vi "SwissSPAD Live_Create HDF5 File.vi"(8 "error in (no error)":errorcluster, 10 "Current Acquisition":i32, 11 "Current Data Set":i32) -> (0 "Error Out":errorcluster, 1 "Notebook Message":string, 2 "# Image Sets":u32, 3 "# Datasets in Series":i32, 5 "Gate Image Data Q Name":string)   [LabVIEW 2021]
uses:
  SwissSPAD Live_Settings List.ctl
  SwissSPAD Live_File Information.ctl
  <vilib>/addons/h5labview2/file/H5Fmode.ctl
  SwissSPAD Live_SSx PCB Version.ctl
  SwissSPAD Live_SS2 DAQ Parameters 3.ctl
  SwissSPAD Live_SS2 Gate Definition.ctl
  SwissSPAD Live_SS3 DAQ Parameters.ctl
  SwissSPAD Live_SS3 Gate Definition.ctl
  SS3 Gate Width Definition Mode.ctl
  <vilib>/Utility/error.llb/Error Cluster From Error Code.vi
  SwissSPAD Live_Globals.vi
  <vilib>/ErrorRing/Error Ring.xnode
  <vilib>/addons/h5labview2/file/H5F.lvlib
  Variant/Variant to Data/Variant to Data.lvlib
panel:
  out "File Folder":path
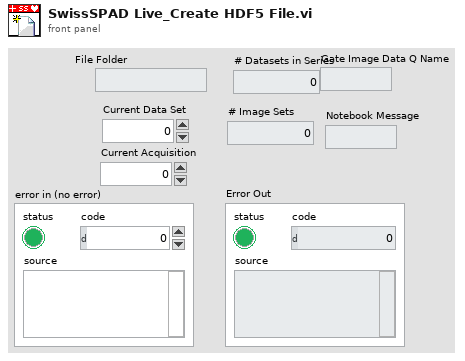
[diagram p1: front panel]
types:
  T1 = typedef "SwissSPAD Live_Settings List.ctl" = enum16{"FPGA:Bottom Half", "FPGA:Top Half", "FPGA:Bottom Bitfile Path", "FPGA:Top Bitfile Path", "FPGA:Bottom Bitstream Version", "FPGA:Top Bitstream Version", "FPGA:Auto Reset FPGA", "FPGA:Bottom FPGA Serial Number", "FPGA:Top FPGA Serial Number", "FPGA:Detector PCB Version", "Acquisition Parameters:Microlens", "Acquisition Parameters:SS2 DAQ Parameters", "Acquisition Parameters:Gate Configuration Array", "Acquisition Parameters:SS3 DAQ Parameters", "Acquisition Parameters:Buffer Size (# 8-bit Gates)", "File Information:File Information", "File Information:# Datasets in Series", "File Information:Scrambled File Flag", "File Information:SS3 Gate Slip Correction", "File Information:SS3 Hot Pixel Mismatch Detection", "File Information:Delay between Datasets", "File Information:Save Sum of All Gates Preview", "Image Parameters:Image ROI Information", "Image Parameters:Image Binning Options", "Image Parameters:SS3 Displayed Image", "Image Parameters:Image Display Options", "Image Parameters:Use Histogram Cursors", "Image Parameter:FPGA Data to Display", "UI Settings:Histogram Bins Number", "UI Settings:Histogram Bin Size", "UI Settings:Use Image Display Options", "UI Settings:Verbose Settings", "UI Settings:Verbose Saving"}
  T2 = typedef "SwissSPAD Live_SSx PCB Version.ctl" = enum16{"unknown", "SS2 PCB1", "SS2 PCB2", "SS3 PCB1"}
  T3 = typedef "H5F.lvlib/H5Fmode.ctl" = enum16{"read-only", "read-write", "overwrite", "create new", "open or create"}
  T4 = typedef "SwissSPAD Live_File Information.ctl" = cluster{"File Folder":path, "File Name":string, "File Index":u32, "Author":string, "Sample":string, "Compression":bool, "Compression Level":u8}
  T5 = typedef "SwissSPAD Live_SS2 DAQ Parameters 3.ctl" = cluster{"10 bits":bool, "# Exposure Sequences":u32, "# 1-bit Frame per Gate":u32, "Gate Shift":u32, "# Gates per Set":u32, "# Sets":u32, "Laser Period":dbl[unit], "Sync Period":dbl[unit], "Gate Offset":u32, "Auto-adjust Gate Offset":bool, "Gate Definition":T6, "Reversed Shift":bool}
  T6 = typedef "SwissSPAD Live_SS2 Gate Definition.ctl" = cluster{"gs_psincdec_0":u32, "gs_psincdec_1":u32, "gs_psincdec_2":u32, "gs_psincdec_3":u32, "gs_no_shift_adj_1":u32, "gs_no_shift_adj_2":u32, "gs_no_shift_adj_3":u32}
  T7 = typedef "SwissSPAD Live_SS3 DAQ Parameters.ctl" = cluster{"10 bits":bool, "# Exposure Sequences":u32, "# 1-bit Frame per Gate":u32, "Gate Shift":u32, "# Gate Pairs per Set":u32, "# Sets":u32, "Laser Period":dbl[unit], "Sync Period":dbl[unit], "Gate Offset":u32, "Auto-adjust Gate Offset":bool, "Gate Definition":T8, "Gate Width (ns)":dbl, "Reversed Shift":bool, "Intensity Mode":bool, "Gate Definition Mode":T9}
  T8 = typedef "SwissSPAD Live_SS3 Gate Definition.ctl" = cluster{"gs_psincdec_0":u32, "gs_psincdec_1":u32, "gs_no_shift_adj_1":u32, "gate_adj_2":u32}
  T9 = typedef "SS3 Gate Width Definition Mode.ctl" = enum32{"Item 0", "Item 1"}
  T10 = typedef "hid_t.ctl" = i32
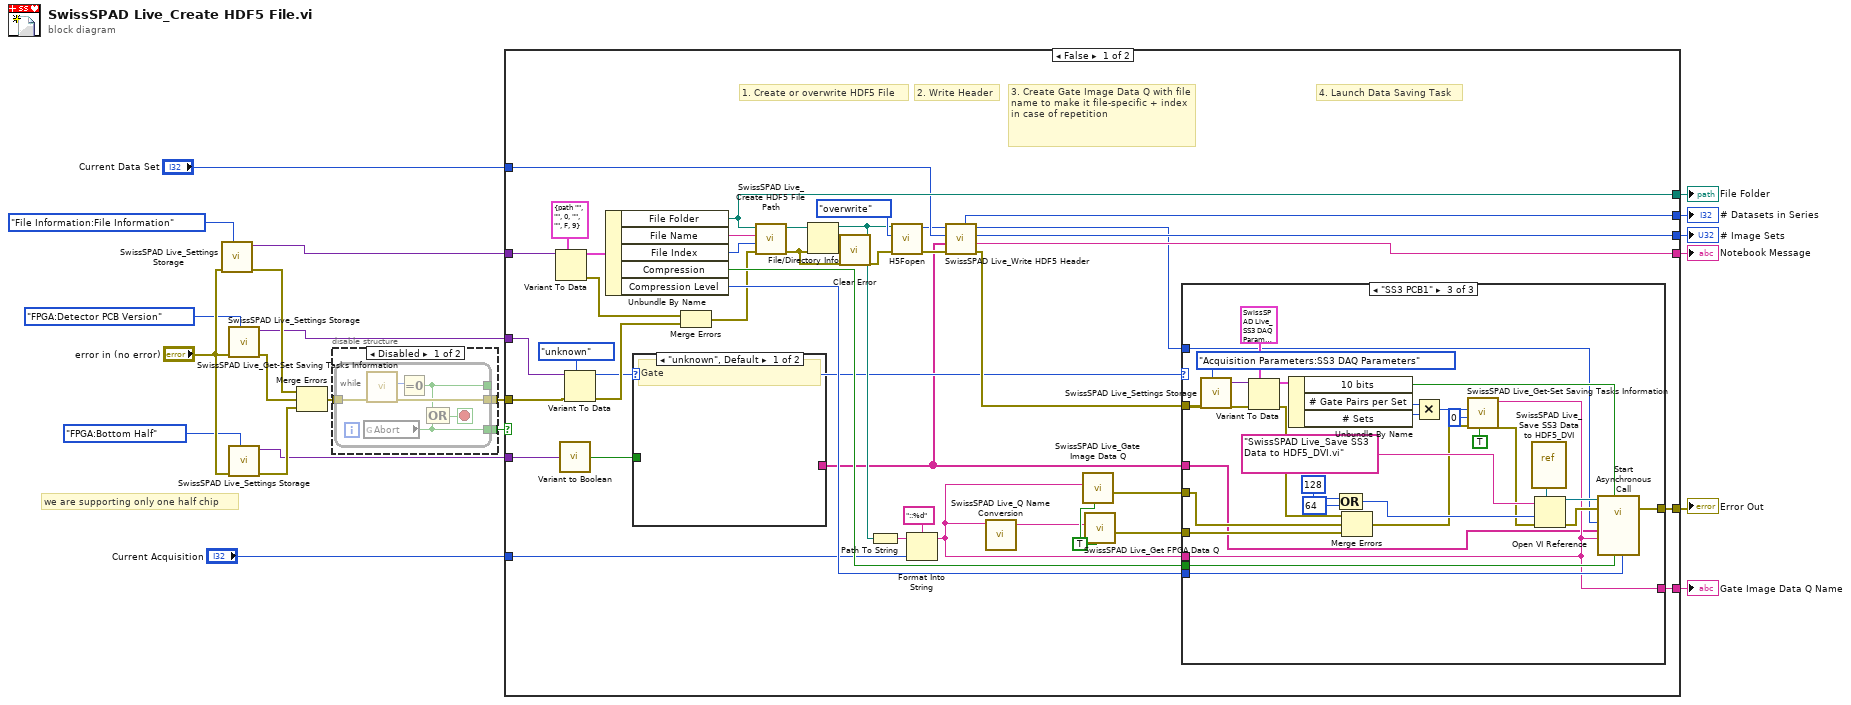
[diagram p0: block diagram]
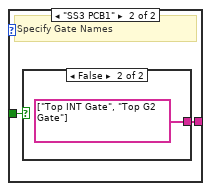
[diagram p3: hidden frame]
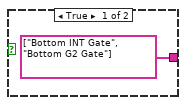
[diagram p4: hidden frame]
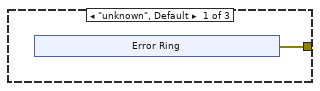
[diagram p5: hidden frame]
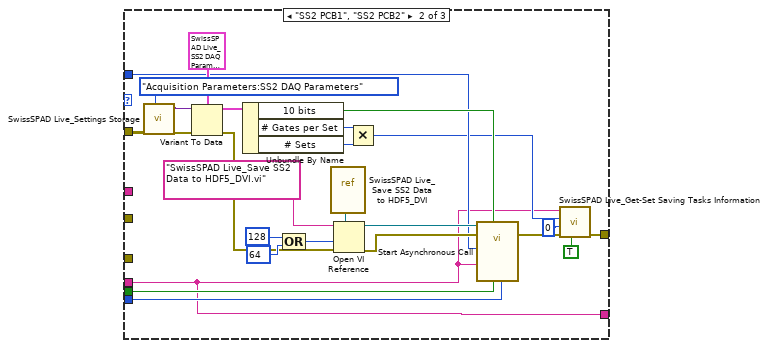
[diagram p6: hidden frame]
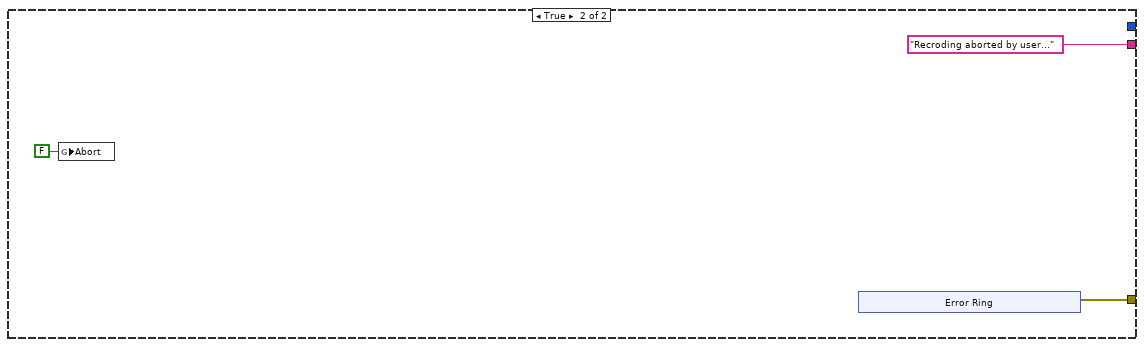
[diagram p7: hidden frame]
diagram:
  # "we are supporting only one half chip"
  n1 = call "SwissSPAD Live_Settings Storage.vi"("Settings List"=SwissSPAD_Live_Settings_List."File Information:File Information", "Error In"="error in (no error)") -> ("Error Out"=w21:errorcluster, "Variant Data out"=w3:variant)  [unwired: 8 in]
  n2 = call "SwissSPAD Live_Settings Storage.vi"("Settings List"=SwissSPAD_Live_Settings_List."FPGA:Detector PCB Version", "Error In"="error in (no error)") -> ("Error Out"=w11:errorcluster, "Variant Data out"=w2:variant)  [unwired: 8 in]
  n3 = call "SwissSPAD Live_Settings Storage.vi"("Settings List"=SwissSPAD_Live_Settings_List."FPGA:Bottom Half", "Error In"="error in (no error)") -> ("Error Out"=w10:errorcluster, "Variant Data out"=w1:variant)  [unwired: 8 in]
  n4 = Merge Errors(w21, w11, w10) -> (w9:errorcluster)
  n5 = disable-structure shown="Disabled" {
    disable-tunnel: w9 -> [w24 w31]
    disable-tunnel: [w23 _] -> w8
    disable-tunnel: [w22 w31] -> w7
    frame Disabled {
      n6 = while {
        tunnel: w24 -> [w30]
        tunnel: [w27] -> w22
        tunnel: [w26] -> _
        tunnel: [w25] -> w23
        stop <- w28 stop-if-true
        n7 = global read "SwissSPAD Live_Globals.vi" "Abort"() -> (w25:bool)
        n8 = call "SwissSPAD Live_Get-Set Saving Tasks Information.vi"("error in (no error)"=w30) -> ("error out"=w27:errorcluster, "# Saving Tasks"=w29:i32)  [unwired: 7 in, 2 out]
        n9 = Equal To 0?(x=w29) -> (x = 0?=w26:bool)
        n10 = Compound Arithmetic op=OR(w26, w25) -> (w28:bool)
      }
    }
    frame Enabled {
    }
  }
  n11 = case shown="False" w8 {
    tunnel: w3 -> [w72 _]
    tunnel: [w69 _] -> w20
    tunnel: [w66 _] -> w19
    tunnel: [w65 "Recroding aborted by user..." ("Notebook Message")] -> w18
    tunnel: [w64 _] -> w17
    tunnel: "Current Data Set" -> [w63 _]
    tunnel: [w62 w139] -> w15
    tunnel: [w58 _] -> w14
    tunnel: w2 -> [w51 _]
    tunnel: "Current Acquisition" -> [w43 _]
    tunnel: w1 -> [w36 _]
    tunnel: w7 -> [w32 _]
    frame False {
      w41 = TRUE ("create if not found? (T)")
      # "4. Launch Data Saving Task"
      # "3. Create Gate Image Data Q with file name to make it file-specific + index in case of repetition"
      # "2. Write Header"
      # "1. Create or overwrite HDF5 File"
      n12 = Variant To Data(type=T4 {"File Folder"=path "", "File Name"="", "File Index"=0, "Author"="", "Sample"="", "Compression"=FALSE, "Compression Level"=9} ("File Information"), Variant=w72) -> (data=w70:T4, error out=w67:errorcluster)  [unwired: 1 in]
      n13 = call "Variant to Boolean.vi"("Variant"=w36) -> ("Value"=w35:bool)  [unwired: 8 in]
      n14 = Variant To Data(error in=w32, type=SwissSPAD_Live_SSx_PCB_Version."unknown" ("Detector PCB Version"), Variant=w51) -> (data=w34:T2, error out=w47:errorcluster)
      n15 = Unbundle By Name(w70) -> ("File Folder"=w69:path, "File Name"=w61:string, "File Index"=w68:u32, "Compression"=w57:bool, "Compression Level"=w56:u8)
      n16 = case shown="\"unknown\", Default" w34 {
        tunnel: w35 -> [_ w74]
        tunnel: [_ w73] -> w33
        frame "unknown", Default {
          # "Gate"
        }
        frame "SS3 PCB1" {
          # "Specify Gate Names"
          n17 = case shown="False" w74 {
            tunnel: [string[] ["Bottom INT Gate", "Bottom G2 Gate"] string[] ["Top INT Gate", "Top G2 Gate"]] -> w73
            frame True {
            }
            frame False {
            }
          }
        }
      }
      n18 = Merge Errors(w67, w47) -> (w48:errorcluster)
      n19 = call "SwissSPAD Live_Create HDF5 File Path.vi"("error in (no error)"=w48, "File Index"=w68, "File Name"=w61, "File Folder"=w69) -> ("error out"=w59:errorcluster, "File path"=w60:path)  [unwired: 6 in]
      n20 = File/Directory Info(path=w60, error in=w59) -> (path out=w45:path, error out=w46:errorcluster)  [unwired: 5 out]
      n21 = call "Clear Error.vi"("Error In"=w46) -> ()  [unwired: 8 in, 1 out]
      n22 = Path To String(path=w45) -> (string=w42:string)
      n23 = call <vilib>:"H5Fopen.vi"("error in (no error)"=w59, "mode (read-only)"=H5Fmode."overwrite", "path"=w45) -> ("error out"=w53:errorcluster, "ref out"=w54:T10)  [unwired: 7 in]
      n24 = Format Into String(format string="::%d", initial string=w42, w43) -> (resulting string=w38:string)  [unwired: 1 in, 1 out]
      n25 = call "SwissSPAD Live_Write HDF5 Header.vi"("error in (no error)"=w53, "Gate Names"=w33, "Current Data Set"=w63, "ref in"=w54) -> ("Error Out"=w49:errorcluster, "Notebook Message"=w65:string, "# Image Sets"=w66:u32, "ref out"=w52:T10, "# Datasets in Series"=w64:i32)  [unwired: 3 in]
      n26 = call "SwissSPAD Live_Q Name Conversion.vi"("SwissSPAD Live Gate Data Decode Q Name"=w38) -> ("FPGA Q Name"=w37:string)  [unwired: 10 in]
      n27 = call "SwissSPAD Live_Gate Image Data Q.vi"("create if not found? (T)"=w41, "SwissSPAD Live Gate Image Data Q Name"=w38) -> ("error out"=w39:errorcluster)  [unwired: 7 in, 2 out]
      n28 = call "SwissSPAD Live_Get FPGA Data Q.vi"("create if not found? (T)"=w41, "FPGA Data Q Name"=w37) -> ("error out"=w40:errorcluster)  [unwired: 8 in, 1 out]
      n29 = case shown="\"SS3 PCB1\"" w34 {
        tunnel: [w77 w104 w112] -> w62
        tunnel: w38 -> [_ w84 w116]
        tunnel: [_ w84 w116] -> w58
        tunnel: w57 -> [_ w100 w131]
        tunnel: w56 -> [_ w99 w130]
        tunnel: w52 -> [_ w94 w126]
        tunnel: w49 -> [_ w86 w119]
        tunnel: w40 -> [_ _ w115]
        tunnel: w39 -> [_ _ w114]
        tunnel: w33 -> [_ _ w113]
        frame "unknown", Default {
          n30 = xnode "Error Ring"() -> ("error out"=w77:errorcluster)
        }
        frame "SS2 PCB1", "SS2 PCB2" {
          n31 = call "SwissSPAD Live_Settings Storage.vi"("Settings List"=SwissSPAD_Live_Settings_List."Acquisition Parameters:SS2 DAQ Parameters", "Error In"=w86) -> ("Error Out"=w107:errorcluster, "Variant Data out"=w82:variant)  [unwired: 8 in]
          n32 = Variant To Data(error in=w107, type=T5 {"10 bits"=FALSE, "# Exposure Sequences"=0, "# 1-bit Frame per Gate"=0, "Gate Shift"=0, "# Gates per Set"=0, "# Sets"=1, "Laser Period"=0.0, "Sync Period"=0.0, "Gate Offset"=0, "Auto-adjust Gate Offset"=FALSE, "Gate Definition"={"gs_psincdec_0"=0, "gs_psincdec_1"=0, "gs_psincdec_2"=0, "gs_psincdec_3"=0, "gs_no_shift_adj_1"=0, "gs_no_shift_adj_2"=0, "gs_no_shift_adj_3"=0}, "Reversed Shift"=FALSE} ("SS2 DAQ Parameters"), Variant=w82) -> (data=w105:T5, error out=w85:errorcluster)
          n33 = Unbundle By Name(w105) -> ("10 bits"=w103:bool, "# Gates per Set"=w102:u32, "# Sets"=w101:u32)
          n34 = Compound Arithmetic op=OR(128 ("options"), 64 ("options")) -> (w91:i32)
          n35 = vi-ref "SwissSPAD Live_Save SS2 Data to HDF5_DVI.vi"() -> (w97:refnum<vi>)
          n36 = Open VI Reference(type specifier VI Refnum (for type only)=w97, vi path="SwissSPAD Live_Save SS2 Data to HDF5_DVI.vi" ("Notebook Message"), options=w91, error in (no error)=w85) -> (vi reference=w96:refnum<vi>, error out=w95:errorcluster)  [unwired: 2 in]
          n37 = Multiply(x=w102, y=w101) -> (x*y=w89:u32)
          n38 = call-by-ref "Start Asynchronous Call"(reference=w96, error in=w95, "Compression Level (0-9)"=w99, "Compression"=w100, "10-bit Gate Image"=w103, "File Path::n"=w84, "HDF5 ref"=w94) -> (error out=w90:errorcluster)  [unwired: 6 in, 2 out]
          n39 = call "SwissSPAD Live_Get-Set Saving Tasks Information.vi"("Get (F)/Set"=TRUE, "error in (no error)"=w90, "# New Images Saved (1)"=0 ("# New Images Saved"), "# Images (Total)"=w89, "File Path::n"=w84) -> ("error out"=w104:errorcluster)  [unwired: 3 in, 3 out]
        }
        frame "SS3 PCB1" {
          n40 = call "SwissSPAD Live_Settings Storage.vi"("Settings List"=SwissSPAD_Live_Settings_List."Acquisition Parameters:SS3 DAQ Parameters", "Error In"=w119) -> ("Error Out"=w137:errorcluster, "Variant Data out"=w108:variant)  [unwired: 8 in]
          n41 = Variant To Data(error in=w137, type=T7 {"10 bits"=FALSE, "# Exposure Sequences"=0, "# 1-bit Frame per Gate"=0, "Gate Shift"=0, "# Gate Pairs per Set"=0, "# Sets"=1, "Laser Period"=0.0, "Sync Period"=0.0, "Gate Offset"=0, "Auto-adjust Gate Offset"=FALSE, "Gate Definition"={"gs_psincdec_0"=0, "gs_psincdec_1"=0, "gs_no_shift_adj_1"=0, "gate_adj_2"=0}, "Gate Width (ns)"=0.0, "Reversed Shift"=FALSE, "Intensity Mode"=FALSE, "Gate Definition Mode"=enum."Item 0"} ("SS3 DAQ Parameters"), Variant=w108) -> (data=w135:T7, error out=w118:errorcluster)
          n42 = Unbundle By Name(w135) -> ("10 bits"=w134:bool, "# Gate Pairs per Set"=w133:u32, "# Sets"=w132:u32)
          n43 = Compound Arithmetic op=OR(128 ("options"), 64 ("options")) -> (w123:i32)
          n44 = Merge Errors(w118, w114, w115) -> (w111:errorcluster)
          n45 = Multiply(x=w133, y=w132) -> (x*y=w122:u32)
          n46 = call "SwissSPAD Live_Get-Set Saving Tasks Information.vi"("Get (F)/Set"=TRUE, "error in (no error)"=w111, "# New Images Saved (1)"=0 ("# New Images Saved"), "# Images (Total)"=w122, "File Path::n"=w116) -> ("error out"=w110:errorcluster)  [unwired: 3 in, 3 out]
          n47 = vi-ref "SwissSPAD Live_Save SS3 Data to HDF5_DVI.vi"() -> (w129:refnum<vi>)
          n48 = Open VI Reference(type specifier VI Refnum (for type only)=w129, vi path="SwissSPAD Live_Save SS3 Data to HDF5_DVI.vi" ("Notebook Message"), options=w123, error in (no error)=w110) -> (vi reference=w128:refnum<vi>, error out=w127:errorcluster)  [unwired: 2 in]
          n49 = call-by-ref "Start Asynchronous Call"(reference=w128, error in=w127, "Compression Level (0-9)"=w130, "Compression"=w131, "10-bit Gate Image"=w134, "File Path::n"=w116, "Gate Names"=w113, "HDF5 ref"=w126) -> (error out=w112:errorcluster)  [unwired: 5 in, 2 out]
        }
      }
    }
    frame True {
      n50 = global write "SwissSPAD Live_Globals.vi" "Abort"(FALSE ("Abort")) -> ()
      n51 = xnode "Error Ring"() -> ("error out"=w139:errorcluster)
    }
  }
  "Error Out" <- w15
  "# Image Sets" <- w19
  "File Folder" <- w20
  "Notebook Message" <- w18
  "# Datasets in Series" <- w17
  "Gate Image Data Q Name" <- w14
